vi "FUG_PowerSupply.contents.vi"   [LabVIEW 2014, in "FUG_PowerSupply.lvlib"]
doc: "This is the constructor of a class.\n\nLicense Agreement for this software:\n\nCopyright (C)\nGesellschaft für Schwerionenforschung, GSI\nPlanckstr. 1\n64291 Darmstadt\nGermany\n\nContact: D.Beck@gsi.de \n\nThis program is free software; you can redistribute it and/or modify it under the terms of the \nGNU General Public License as published by the Free Software Foundation; either version 2 of \nthe license, or (at your option) any later version.\n\nThis program is distributed in the hope that it will be useful, but WITHOUT ANY WARRANTY; \nwithout even the implied warranty of MERCHANTABILITY or FITNESS FOR A PARTICULAR PURPOSE. See the GNU General License for more details (http://www.gnu.org).\n\nGesellschaft für Schwerionenforschung, GSI\nPlanckstr. 1, 64291 Darmstadt, Germany\nFor all questions and ideas contact: M.Richter@gsi.de, H.Brand@gsi.de or D.Beck@gsi.de.\nLast update: 16-JUN-2004"
uses:
  FUG_PowerSupply.lvlib
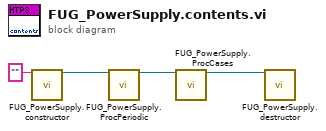
[diagram p0: block diagram]
diagram:
  n1 = call "FUG_PowerSupply.constructor.vi"("name"="") -> ("i ref out"=w4:refnum<vi>)  [unwired: 16 in, 2 out]
  n2 = call "FUG_PowerSupply.ProcPeriodic.vi"("i ref in"=w4) -> ("i ref out"=w3:refnum<vi>)  [unwired: 16 in, 2 out]
  n3 = call "FUG_PowerSupply.ProcCases.vi"("i ref in"=w3) -> ("i ref out"=w2:refnum<vi>)  [unwired: 16 in, 2 out]
  n4 = call "FUG_PowerSupply.destructor.vi"("i ref in"=w2) -> ()  [unwired: 18 in, 1 out]
